vi "SW_Calc_speed.vi"(3 "SG coefficients":T1, 4 "X coord, mm":dbl, 5 "Y coord, mm":dbl, 6 "Time per frame, s":dbl) -> (0 "Mouse speed for TTL detection, mm/s":dbl, 1 "Mouse speed, mm/s":dbl, 2 "Mouse speed for saving, mm/s":string)   [LabVIEW 2018, in "Tracker.lvlib"]
doc: "This VI calculates speed using smoothing of the input noisy data according to Holoborodko' algorithm: http://www.holoborodko.com/pavel/numerical-methods/numerical-derivative/smooth-low-noise-differentiator"
uses:
  Tracker.lvlib
panel:
  in  "Speed smoothing type":u16(ring)=3 items=["None", "Holoborodko 2/5", "Holoborodko 2/7", "Holoborodko 2/11", "Holoborodko 4/7"]
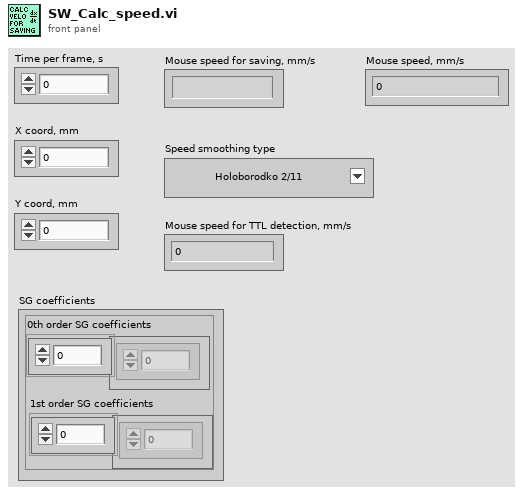
[diagram p1: front panel]
types:
  T1 = cluster{"0th order SG coefficients":dbl[], "1st order SG coefficients":dbl[]}
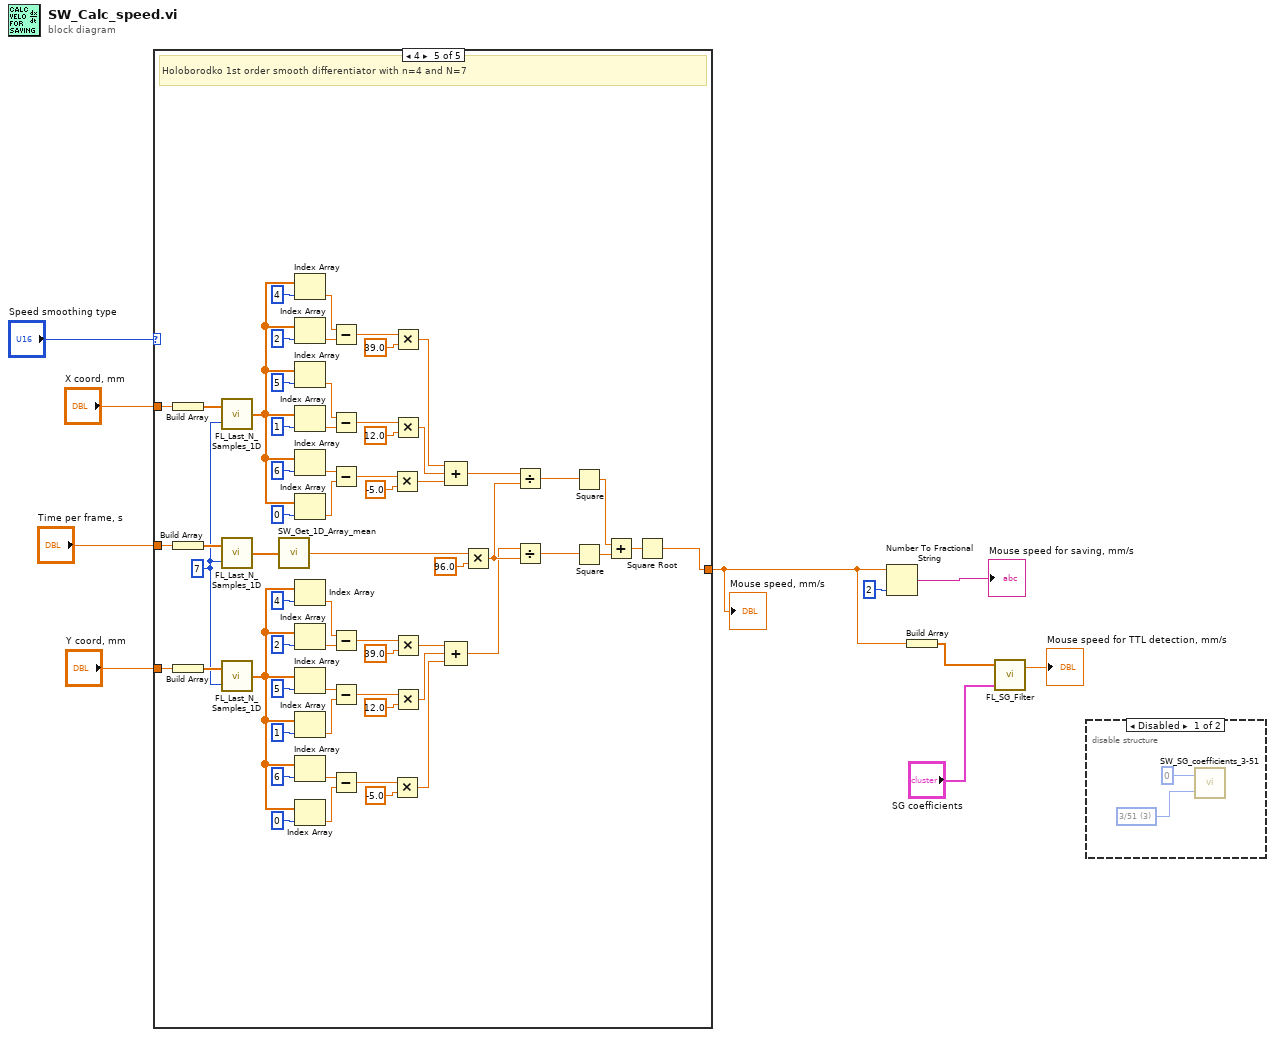
[diagram p0: block diagram]
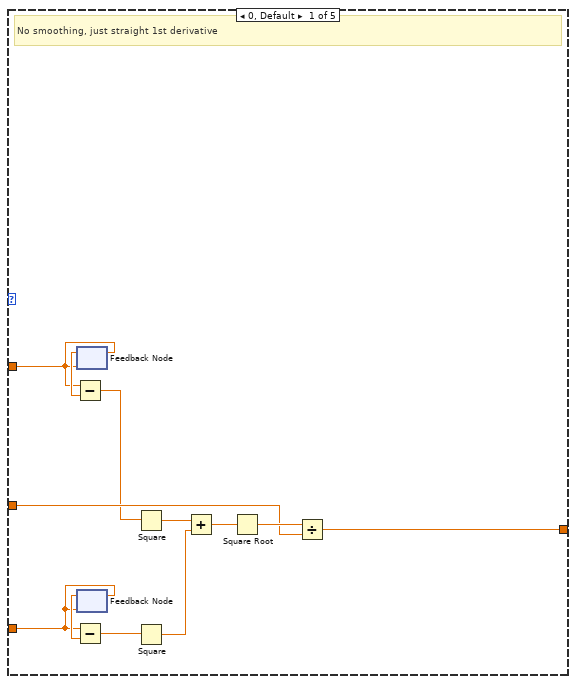
[diagram p3: hidden frame]
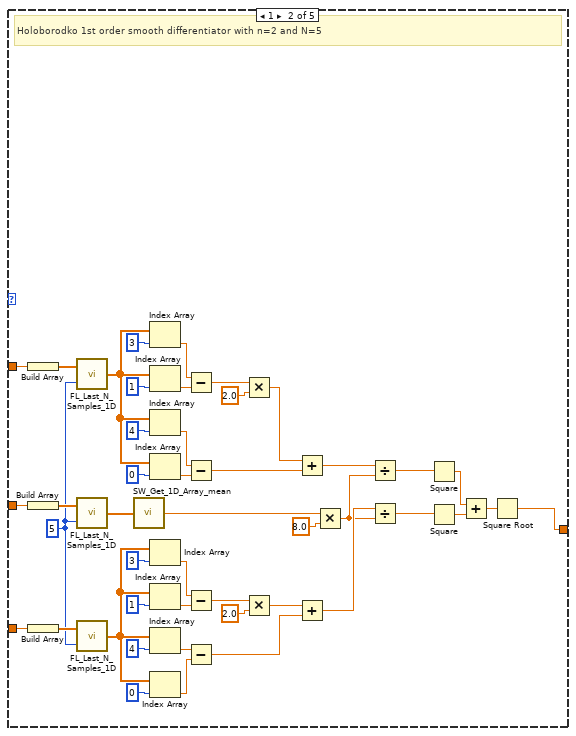
[diagram p4: hidden frame]
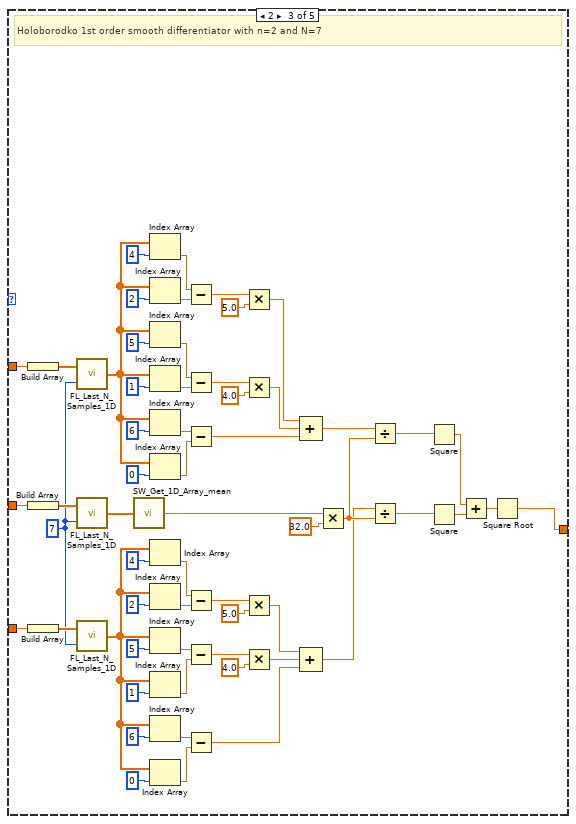
[diagram p5: hidden frame]
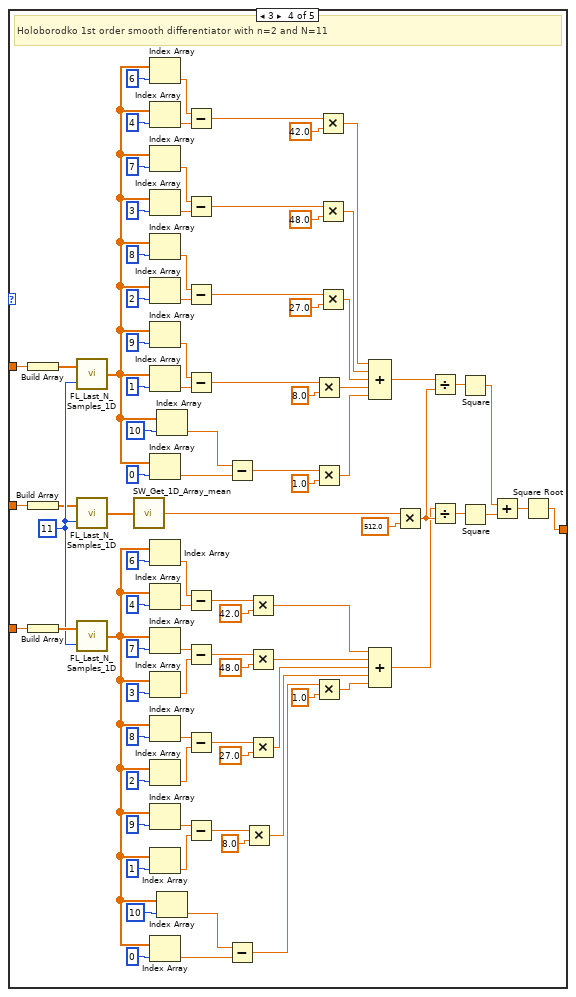
[diagram p6: hidden frame]
diagram:
  n1 = case shown="4" "Speed smoothing type" {
    tunnel: "Time per frame, s" -> [w18 w67 w126 w130 w280]
    tunnel: "Y coord, mm" -> [w12 w63 w122 w215 w276]
    tunnel: "X coord, mm" -> [w14 w62 w121 w214 w275]
    tunnel: [w17 w25 w104 w197 w258] -> w2
    frame 0, Default {
      # "No smoothing, just straight 1st derivative"
      n2 = feedback #1(w14) -> (w15:dbl)
      n3 = Subtract(x=w14, y=w15) -> (x-y=w13:dbl)
      n4 = feedback-in #1(w14) -> ()
      n5 = feedback #2(w12) -> (w16:dbl)
      n6 = Subtract(x=w12, y=w16) -> (x-y=w11:dbl)
      n7 = feedback-in #2(w12) -> ()
      n8 = Square(x=w13) -> (x^2=w21:dbl)
      n9 = Square(x=w11) -> (x^2=w22:dbl)
      n10 = Add(x=w21, y=w22) -> (x+y=w20:dbl)
      n11 = Square Root(x=w20) -> (sqrt(x)=w19:dbl)
      n12 = Divide(x=w19, y=w18) -> (x/y=w17:dbl)
    }
    frame 1 {
      w61 = u32 5 ("BufferLengthSamples")
      # "Holoborodko 1st order smooth differentiator with n=2 and N=5"
      n13 = Build Array(w62) -> (w65:dbl[])
      n14 = Build Array(w67) -> (w66:dbl[])
      n15 = Build Array(w63) -> (w64:dbl[])
      n16 = call "FL_Last_N_Samples_1D.vi"("BufferLengthSamples"=w61, "Input Array"=w65) -> ("Output Array"=w52:dbl[])
      n17 = call "FL_Last_N_Samples_1D.vi"("BufferLengthSamples"=w61, "Input Array"=w66) -> ("Output Array"=w24:dbl[])
      n18 = call "FL_Last_N_Samples_1D.vi"("BufferLengthSamples"=w61, "Input Array"=w64) -> ("Output Array"=w32:dbl[])
      n19 = call "SW_Get_1D_Array_mean.vi"("1D array"=w24) -> ("Mean of 1D Array"=w23:dbl)
      n20 = Index Array(array=w52, index=3) -> (element=w58:dbl)
      n21 = Index Array(array=w52, index=1) -> (element=w57:dbl)
      n22 = Index Array(array=w52, index=4) -> (element=w51:dbl)
      n23 = Index Array(array=w52, index=0) -> (element=w50:dbl)
      n24 = Index Array(array=w32, index=3) -> (element=w35:dbl)
      n25 = Index Array(array=w32, index=1) -> (element=w36:dbl)
      n26 = Index Array(array=w32, index=4) -> (element=w41:dbl)
      n27 = Index Array(array=w32, index=0) -> (element=w42:dbl)
      n28 = Subtract(x=w58, y=w57) -> (x-y=w56:dbl)
      n29 = Subtract(x=w51, y=w50) -> (x-y=w48:dbl)
      n30 = Subtract(x=w35, y=w36) -> (x-y=w37:dbl)
      n31 = Subtract(x=w41, y=w42) -> (x-y=w44:dbl)
      n32 = Multiply(x=w56, y=2.0) -> (x*y=w49:dbl)
      n33 = Multiply(x=w37, y=2.0) -> (x*y=w43:dbl)
      n34 = Add(x=w49, y=w48) -> (x+y=w47:dbl)
      n35 = Add(x=w43, y=w44) -> (x+y=w45:dbl)
      n36 = Multiply(x=w23, y=8.0) -> (x*y=w31:dbl)
      n37 = Divide(x=w47, y=w31) -> (x/y=w28:dbl)
      n38 = Divide(x=w45, y=w31) -> (x/y=w26:dbl)
      n39 = Square(x=w28) -> (x^2=w27:dbl)
      n40 = Square(x=w26) -> (x^2=w29:dbl)
      n41 = Add(x=w27, y=w29) -> (x+y=w30:dbl)
      n42 = Square Root(x=w30) -> (sqrt(x)=w25:dbl)
    }
    frame 2 {
      w120 = u32 7 ("BufferLengthSamples")
      # "Holoborodko 1st order smooth differentiator with n=2 and N=7"
      n43 = Build Array(w121) -> (w124:dbl[])
      n44 = Build Array(w126) -> (w125:dbl[])
      n45 = Build Array(w122) -> (w123:dbl[])
      n46 = call "FL_Last_N_Samples_1D.vi"("BufferLengthSamples"=w120, "Input Array"=w124) -> ("Output Array"=w99:dbl[])
      n47 = call "FL_Last_N_Samples_1D.vi"("BufferLengthSamples"=w120, "Input Array"=w125) -> ("Output Array"=w69:dbl[])
      n48 = call "FL_Last_N_Samples_1D.vi"("BufferLengthSamples"=w120, "Input Array"=w123) -> ("Output Array"=w72:dbl[])
      n49 = call "SW_Get_1D_Array_mean.vi"("1D array"=w69) -> ("Mean of 1D Array"=w68:dbl)
      n50 = Index Array(array=w99, index=4) -> (element=w117:dbl)
      n51 = Index Array(array=w99, index=2) -> (element=w116:dbl)
      n52 = Index Array(array=w99, index=5) -> (element=w113:dbl)
      n53 = Index Array(array=w99, index=1) -> (element=w112:dbl)
      n54 = Index Array(array=w99, index=6) -> (element=w102:dbl)
      n55 = Index Array(array=w99, index=0) -> (element=w103:dbl)
      n56 = Index Array(array=w72, index=4) -> (element=w75:dbl)
      n57 = Index Array(array=w72, index=2) -> (element=w76:dbl)
      n58 = Index Array(array=w72, index=5) -> (element=w79:dbl)
      n59 = Index Array(array=w72, index=1) -> (element=w80:dbl)
      n60 = Index Array(array=w72, index=6) -> (element=w82:dbl)
      n61 = Index Array(array=w72, index=0) -> (element=w81:dbl)
      n62 = Subtract(x=w117, y=w116) -> (x-y=w98:dbl)
      n63 = Subtract(x=w113, y=w112) -> (x-y=w96:dbl)
      n64 = Subtract(x=w102, y=w103) -> (x-y=w94:dbl)
      n65 = Subtract(x=w75, y=w76) -> (x-y=w85:dbl)
      n66 = Subtract(x=w79, y=w80) -> (x-y=w87:dbl)
      n67 = Subtract(x=w82, y=w81) -> (x-y=w89:dbl)
      n68 = Multiply(x=w98, y=5.0) -> (x*y=w92:dbl)
      n69 = Multiply(x=w96, y=4.0) -> (x*y=w93:dbl)
      n70 = Multiply(x=w85, y=5.0) -> (x*y=w91:dbl)
      n71 = Multiply(x=w87, y=4.0) -> (x*y=w90:dbl)
      n72 = Compound Arithmetic op=ADD(w92, w93, w94) -> (w71:dbl)
      n73 = Compound Arithmetic op=ADD(w91, w90, w89) -> (w70:dbl)
      n74 = Multiply(x=w68, y=32.0) -> (x*y=w110:dbl)
      n75 = Divide(x=w71, y=w110) -> (x/y=w107:dbl)
      n76 = Divide(x=w70, y=w110) -> (x/y=w105:dbl)
      n77 = Square(x=w107) -> (x^2=w106:dbl)
      n78 = Square(x=w105) -> (x^2=w108:dbl)
      n79 = Add(x=w106, y=w108) -> (x+y=w109:dbl)
      n80 = Square Root(x=w109) -> (sqrt(x)=w104:dbl)
    }
    frame 3 {
      w213 = u32 11 ("BufferLengthSamples")
      # "Holoborodko 1st order smooth differentiator with n=2 and N=11"
      n81 = Build Array(w214) -> (w217:dbl[])
      n82 = Build Array(w130) -> (w129:dbl[])
      n83 = Build Array(w215) -> (w216:dbl[])
      n84 = call "FL_Last_N_Samples_1D.vi"("BufferLengthSamples"=w213, "Input Array"=w217) -> ("Output Array"=w170:dbl[])
      n85 = call "FL_Last_N_Samples_1D.vi"("BufferLengthSamples"=w213, "Input Array"=w129) -> ("Output Array"=w128:dbl[])
      n86 = call "FL_Last_N_Samples_1D.vi"("BufferLengthSamples"=w213, "Input Array"=w216) -> ("Output Array"=w132:dbl[])
      n87 = call "SW_Get_1D_Array_mean.vi"("1D array"=w128) -> ("Mean of 1D Array"=w127:dbl)
      n88 = Index Array(array=w170, index=6) -> (element=w210:dbl)
      n89 = Index Array(array=w170, index=4) -> (element=w209:dbl)
      n90 = Index Array(array=w170, index=7) -> (element=w206:dbl)
      n91 = Index Array(array=w170, index=3) -> (element=w205:dbl)
      n92 = Index Array(array=w170, index=8) -> (element=w195:dbl)
      n93 = Index Array(array=w170, index=2) -> (element=w196:dbl)
      n94 = Index Array(array=w170, index=9) -> (element=w178:dbl)
      n95 = Index Array(array=w170, index=1) -> (element=w177:dbl)
      n96 = Index Array(array=w170, index=0) -> (element=w176:dbl)
      n97 = Index Array(array=w132, index=6) -> (element=w135:dbl)
      n98 = Index Array(array=w132, index=4) -> (element=w136:dbl)
      n99 = Index Array(array=w132, index=7) -> (element=w139:dbl)
      n100 = Index Array(array=w132, index=3) -> (element=w140:dbl)
      n101 = Index Array(array=w132, index=8) -> (element=w142:dbl)
      n102 = Index Array(array=w132, index=2) -> (element=w141:dbl)
      n103 = Index Array(array=w132, index=9) -> (element=w158:dbl)
      n104 = Index Array(array=w132, index=1) -> (element=w159:dbl)
      n105 = Index Array(array=w132, index=0) -> (element=w160:dbl)
      n106 = Index Array(array=w170, index=10) -> (element=w175:dbl)
      n107 = Index Array(array=w132, index=10) -> (element=w161:dbl)
      n108 = Subtract(x=w210, y=w209) -> (x-y=w192:dbl)
      n109 = Subtract(x=w206, y=w205) -> (x-y=w190:dbl)
      n110 = Subtract(x=w195, y=w196) -> (x-y=w188:dbl)
      n111 = Subtract(x=w178, y=w177) -> (x-y=w181:dbl)
      n112 = Subtract(x=w135, y=w136) -> (x-y=w145:dbl)
      n113 = Subtract(x=w139, y=w140) -> (x-y=w147:dbl)
      n114 = Subtract(x=w142, y=w141) -> (x-y=w149:dbl)
      n115 = Subtract(x=w158, y=w159) -> (x-y=w155:dbl)
      n116 = Subtract(x=w175, y=w176) -> (x-y=w172:dbl)
      n117 = Subtract(x=w161, y=w160) -> (x-y=w164:dbl)
      n118 = Multiply(x=w155, y=8.0) -> (x*y=w166:dbl)
      n119 = Multiply(x=w145, y=42.0) -> (x*y=w151:dbl)
      n120 = Multiply(x=w147, y=48.0) -> (x*y=w150:dbl)
      n121 = Multiply(x=w149, y=27.0) -> (x*y=w152:dbl)
      n122 = Multiply(x=w181, y=8.0) -> (x*y=w169:dbl)
      n123 = Multiply(x=w172, y=1.0) -> (x*y=w168:dbl)
      n124 = Multiply(x=w164, y=1.0) -> (x*y=w167:dbl)
      n125 = Multiply(x=w192, y=42.0) -> (x*y=w186:dbl)
      n126 = Multiply(x=w190, y=48.0) -> (x*y=w187:dbl)
      n127 = Multiply(x=w188, y=27.0) -> (x*y=w184:dbl)
      n128 = Compound Arithmetic op=ADD(w186, w187, w184, w169, w168) -> (w185:dbl)
      n129 = Compound Arithmetic op=ADD(w151, w150, w152, w166, w167) -> (w131:dbl)
      n130 = Multiply(x=w127, y=512.0) -> (x*y=w203:dbl)
      n131 = Divide(x=w185, y=w203) -> (x/y=w200:dbl)
      n132 = Divide(x=w131, y=w203) -> (x/y=w198:dbl)
      n133 = Square(x=w200) -> (x^2=w199:dbl)
      n134 = Square(x=w198) -> (x^2=w201:dbl)
      n135 = Add(x=w199, y=w201) -> (x+y=w202:dbl)
      n136 = Square Root(x=w202) -> (sqrt(x)=w197:dbl)
    }
    frame 4 {
      w274 = u32 7 ("BufferLengthSamples")
      # "Holoborodko 1st order smooth differentiator with n=4 and N=7"
      n137 = Build Array(w275) -> (w278:dbl[])
      n138 = Build Array(w280) -> (w279:dbl[])
      n139 = Build Array(w276) -> (w277:dbl[])
      n140 = call "FL_Last_N_Samples_1D.vi"("BufferLengthSamples"=w274, "Input Array"=w278) -> ("Output Array"=w253:dbl[])
      n141 = call "FL_Last_N_Samples_1D.vi"("BufferLengthSamples"=w274, "Input Array"=w279) -> ("Output Array"=w219:dbl[])
      n142 = call "FL_Last_N_Samples_1D.vi"("BufferLengthSamples"=w274, "Input Array"=w277) -> ("Output Array"=w226:dbl[])
      n143 = call "SW_Get_1D_Array_mean.vi"("1D array"=w219) -> ("Mean of 1D Array"=w218:dbl)
      n144 = Index Array(array=w253, index=4) -> (element=w271:dbl)
      n145 = Index Array(array=w253, index=2) -> (element=w270:dbl)
      n146 = Index Array(array=w253, index=5) -> (element=w267:dbl)
      n147 = Index Array(array=w253, index=1) -> (element=w266:dbl)
      n148 = Index Array(array=w253, index=6) -> (element=w256:dbl)
      n149 = Index Array(array=w253, index=0) -> (element=w257:dbl)
      n150 = Index Array(array=w226, index=4) -> (element=w229:dbl)
      n151 = Index Array(array=w226, index=2) -> (element=w230:dbl)
      n152 = Index Array(array=w226, index=5) -> (element=w233:dbl)
      n153 = Index Array(array=w226, index=1) -> (element=w234:dbl)
      n154 = Index Array(array=w226, index=6) -> (element=w236:dbl)
      n155 = Index Array(array=w226, index=0) -> (element=w235:dbl)
      n156 = Subtract(x=w271, y=w270) -> (x-y=w252:dbl)
      n157 = Subtract(x=w267, y=w266) -> (x-y=w250:dbl)
      n158 = Subtract(x=w256, y=w257) -> (x-y=w248:dbl)
      n159 = Subtract(x=w229, y=w230) -> (x-y=w239:dbl)
      n160 = Subtract(x=w233, y=w234) -> (x-y=w241:dbl)
      n161 = Subtract(x=w236, y=w235) -> (x-y=w243:dbl)
      n162 = Multiply(x=w248, y=-5.0) -> (x*y=w223:dbl)
      n163 = Multiply(x=w243, y=-5.0) -> (x*y=w221:dbl)
      n164 = Multiply(x=w252, y=39.0) -> (x*y=w246:dbl)
      n165 = Multiply(x=w250, y=12.0) -> (x*y=w247:dbl)
      n166 = Multiply(x=w239, y=39.0) -> (x*y=w245:dbl)
      n167 = Multiply(x=w241, y=12.0) -> (x*y=w244:dbl)
      n168 = Compound Arithmetic op=ADD(w246, w247, w223) -> (w225:dbl)
      n169 = Compound Arithmetic op=ADD(w245, w244, w221) -> (w224:dbl)
      n170 = Multiply(x=w218, y=96.0) -> (x*y=w264:dbl)
      n171 = Divide(x=w225, y=w264) -> (x/y=w261:dbl)
      n172 = Divide(x=w224, y=w264) -> (x/y=w259:dbl)
      n173 = Square(x=w261) -> (x^2=w260:dbl)
      n174 = Square(x=w259) -> (x^2=w262:dbl)
      n175 = Add(x=w260, y=w262) -> (x+y=w263:dbl)
      n176 = Square Root(x=w263) -> (sqrt(x)=w258:dbl)
    }
  }
  "Mouse speed, mm/s" <- w2
  n177 = Number To Fractional String(number=w2, precision (6)=i16 2) -> (F-format string=→"Mouse speed for saving, mm/s":string)  [unwired: 2 in]
  n178 = Build Array(w2) -> (w3:dbl[])
  n179 = call "FL_SG_Filter.vi"("SG coefficients"="SG coefficients", "Input array of data"=w3) -> ("Filtered data, 0 order"=→"Mouse speed for TTL detection, mm/s":dbl)  [unwired: 2 in]
  n180 = disable-structure shown="Disabled" {
    frame Disabled {
      w281 = u16 3 items=["3/5", "3/11", "3/31", "3/51"] ("Select filter length")
      n181 = call "SW_SG_coefficients_3-51.vi"("Select filter length"=w281, "Point of interest (can be used for extrapolation)"=0) -> ()  [unwired: 1 in, 1 out]
    }
    frame Enabled {
    }
  }
